vi "Generate New File Name.vi"(8 "error in (no error)":errorcluster, 11 "Logger in":refnum<class "Logger.lvclass">) -> (0 "error out":errorcluster, 3 "Logger out":refnum<class "Logger.lvclass">)   [LabVIEW 2026, in "Logger.lvlib" / "Logger.lvclass"]
uses:
  Logger.lvclass
  Logger.lvclass/Logger.ctl
  config/Logger Configuration.lvclass/Logger Configuration.ctl
  config/Read Logging Settings.vi
  recovery/packages/oglib_file-4.0.1.22-8A89CE420A/File Group 0/user.lib/_OpenG.lib/file/file.llb/Convert File Extension (String)__ogtk.vi
  config/Logger Configuration.lvclass
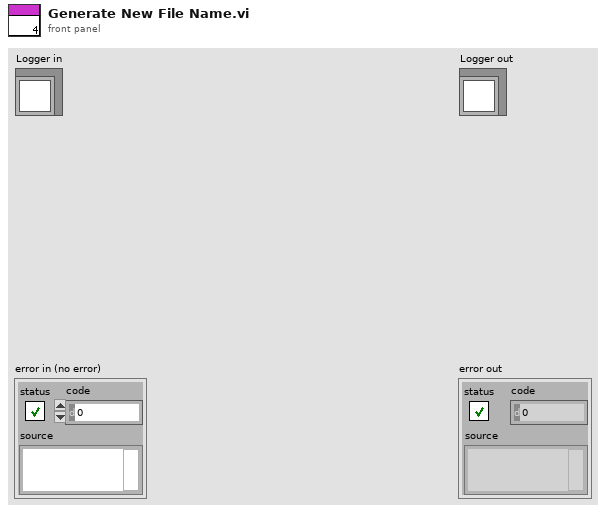
[diagram p1: front panel]
types:
  T1 = cluster{"File Name":string, "Upload Files to SystemLink Server":bool, "Max Samples Per File":i32, "Folder Location":path, "Logging":bool}
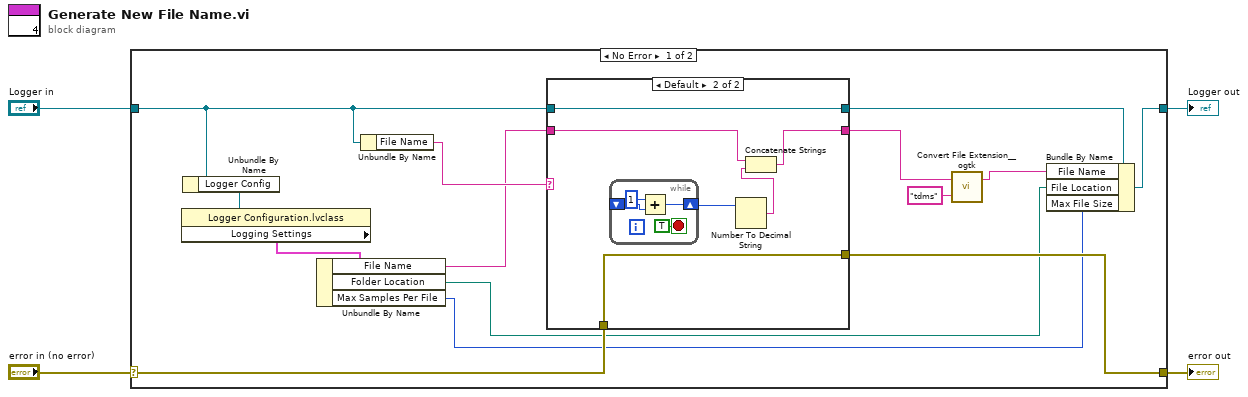
[diagram p0: block diagram]
diagram:
  n1 = case shown="No Error" "error in (no error)" {
    selector: "error in (no error)" -> [w18 w33]
    tunnel: [w17 w33] -> w3
    tunnel: [w15 w32] -> w1
    tunnel: "Logger in" -> [w9 w32]
    frame No Error {
      n2 = Unbundle By Name(w9) -> ("Logger Config"=w11:refnum<class "Logger Configuration.lvclass">)
      n3 = property class="Logger Configuration.lvclass"(reference=w11) -> ("Logging Settings"=w10:T1)  [unwired: 1 in, 2 out]
      n4 = Unbundle By Name(w10) -> ("File Name"=w7:string, "Folder Location"=w6:path, "Max Samples Per File"=w5:i32)
      n5 = Unbundle By Name(w9) -> ("File Name"=w8:string)
      n6 = case shown="Default" w8 {
        tunnel: w18 -> [w21 w27]
        tunnel: [w20 w26] -> w16
        tunnel: [w21 w27] -> w17
        tunnel: w9 -> [w20 w26]
        tunnel: [w19 w23] -> w13
        tunnel: w7 -> [w19 w22]
        frame "" {
        }
        frame Default {
          n7 = while {
            shift-right: [w28] -> w25
            shift-left: _ -> [w30]
            stop <- TRUE stop-if-true
            n8 = Add(x=1, y=w30) -> (x+y=w28:i32)
          }
          n9 = Number To Decimal String(number=w25) -> (decimal integer string=w24:string)  [unwired: 1 in]
          n10 = Concatenate Strings(w22, w24) -> (w23:string)
        }
      }
      n11 = call-poly "Convert File Extension__ogtk.vi"("new ending (none)"="tdms", "file name"=w13) -> ("new filename"=w12:string)  [unwired: 1 out]
      n12 = Bundle By Name(cluster=w16, "File Name"=w12, "File Location"=w6, "Max File Size"=w5) -> (w15:refnum<class "Logger.lvclass">)
    }
    frame Error {
    }
  }
  "error out" <- w3
  "Logger out" <- w1
